vi "Configure Output.vi"(8 "error in (no error)":errorcluster, 9 "Output Power On State (0: Reset)":i32(ring) items=["Reset", "Recall Location 0"], 10 "Enable Output (F: Disable)":bool, 11 "VISA resource name":refnum<visa-resource-name>) -> (0 "error out":errorcluster, 3 "VISA resource name out":refnum<visa-resource-name>)   [LabVIEW 2017, in "Keysight N8900 Series.lvlib"]
doc: "Configures the output."
uses:
  Keysight N8900 Series.lvlib
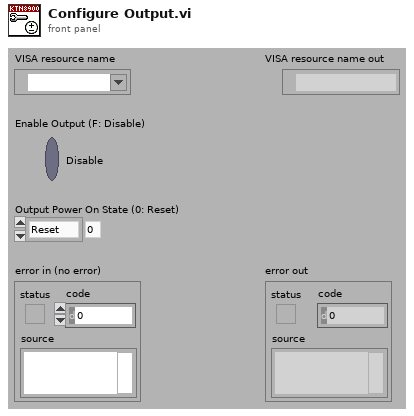
[diagram p1: front panel]
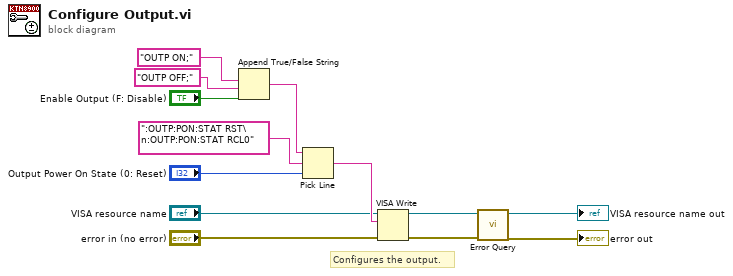
[diagram p0: block diagram]
diagram:
  # "Configures the output."
  n1 = Append True/False String(1:"Enable Output (F: Disable)", 2:"OUTP OFF;", 3:"OUTP ON;") -> (0:w8:string)  [unwired: 1 in]
  n2 = Pick Line(string ("")=w8, multi-line string=":OUTP:PON:STAT RST\n:OUTP:PON:STAT RCL0", line index="Output Power On State (0: Reset)") -> (output string=w7:string)
  n3 = VISA Write(VISA resource name="VISA resource name", write buffer=w7, error in (no error)="error in (no error)") -> (VISA resource name out=w4:refnum<visa-resource-name>, error out=w3:errorcluster)  [unwired: 1 out]
  n4 = call "Error Query.vi"("error in (no error)"=w3, "VISA resource name"=w4) -> ("error out"=→"error out":errorcluster, "VISA resource name out"=→"VISA resource name out":refnum<visa-resource-name>)  [unwired: 6 in, 2 out]
